vi "Offset.vi"(8 "error in (no error)":errorcluster, 11 "IV in":refnum<class "IV.lvclass">) -> (0 "error out":errorcluster, 3 "IV out":refnum<class "IV.lvclass">)   [LabVIEW 2018, in "IV.lvclass"]
uses:
  IV.lvclass
  IV.lvclass/IV.ctl
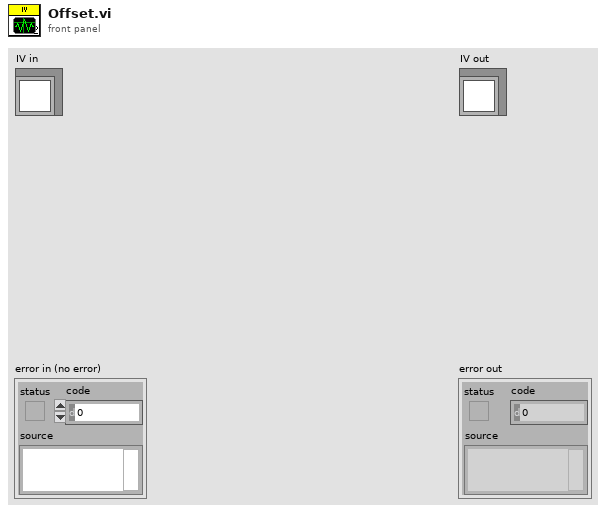
[diagram p1: front panel]
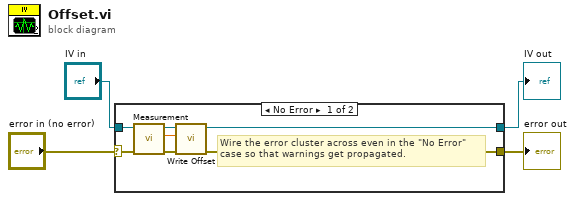
[diagram p0: block diagram]
diagram:
  n1 = case shown="No Error" "error in (no error)" {
    selector: "error in (no error)" -> [w8 w13]
    tunnel: [w5 w13] -> w3
    tunnel: [w6 w12] -> w1
    tunnel: "IV in" -> [w7 w12]
    frame No Error {
      # "Wire the error cluster across even in the \"No Error\"\ncase so that warnings get propagated."
      n2 = call-dynamic "Measurement.vi"("error in (no error)"=w8, "IV in"=w7) -> ("error out"=w9:errorcluster, "Result"=w10:dbl, "IV out"=w11:refnum<class "IV.lvclass">)  [unwired: 6 in, 1 out]
      n3 = call "Write Offset.vi"("error in (no error)"=w9, "Offset"=w10, "IV in"=w11) -> ("error out"=w5:errorcluster, "IV out"=w6:refnum<class "IV.lvclass">)  [unwired: 7 in]
    }
    frame Error {
    }
  }
  "error out" <- w3
  "IV out" <- w1
